vi "Next Column (name).vi"(8 "error in (no error)":errorcluster, 10 "parameter name":string, 11 "SQL Statement in":refnum<class "SQL Statement.lvclass">) -> (0 "error out":errorcluster, 3 "SQL Statement out":refnum<class "SQL Statement.lvclass">)   [LabVIEW 2023]
doc: "Sets the next parameter to be bound to, by its name. Name formats are ?NNN, :VVV, @VVV or $VVV where NNN are numeric digits and VVV are alphanumeric characters. Names are specified in the SQL statement."
uses:
  SQL Statement.lvclass
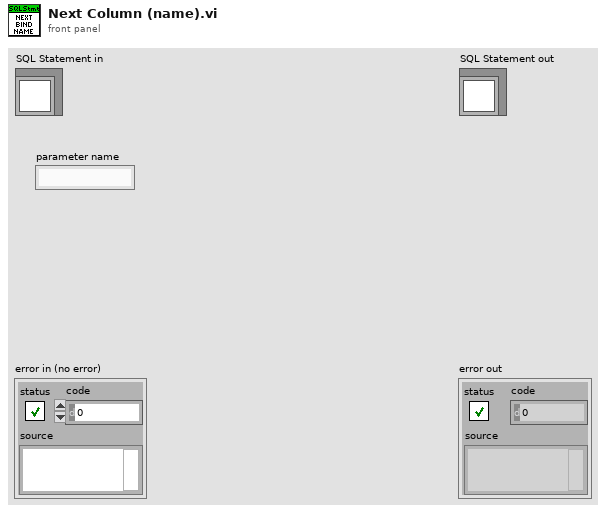
[diagram p1: front panel]
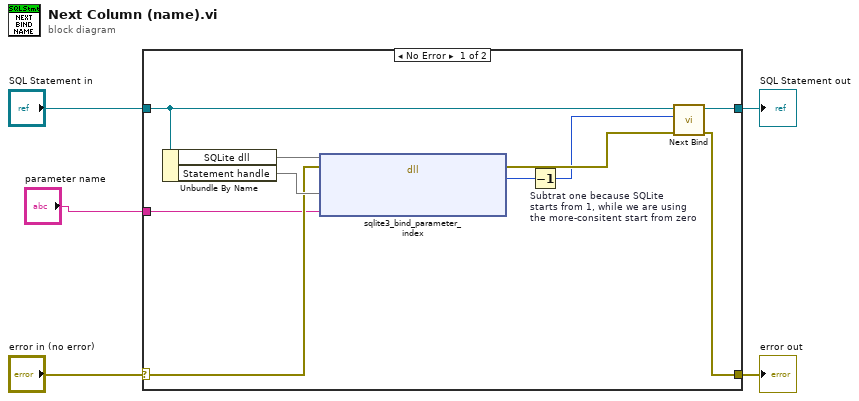
[diagram p0: block diagram]
diagram:
  n1 = case shown="No Error" "error in (no error)" {
    selector: "error in (no error)" -> [w13 w17]
    tunnel: [w7 w17] -> w4
    tunnel: [w10 w16] -> w2
    tunnel: "SQL Statement in" -> [w11 w16]
    tunnel: "parameter name" -> [w12 _]
    frame No Error {
      n2 = Unbundle By Name(w11) -> ("SQLite dll"=w15, "Statement handle"=w14)
      n3 = dll-call lib="C:/LabVIEW_JDP/Support/SQLite/sqlite3.dll" fn="sqlite3_bind_parameter_index"(path in=w15, error in=w13, "Statement"=w14, "name"=w12) -> (error out=w8:errorcluster, "Paramter index"=w9:i32)  [unwired: 3 in, 1 out]
      n4 = Decrement "Subtrat one because SQLite\nstarts from 1, while we are using\nthe more-consitent start from zero"(x=w9) -> (x-1=w6:i32)
      n5 = call "Next Bind.vi"("error in (no error)"=w8, "Next Bind"=w6, "SQL Statement in"=w11) -> ("error out"=w7:errorcluster, "SQL Statement out"=w10:refnum<class "SQL Statement.lvclass">)  [unwired: 7 in]
    }
    frame Error {
    }
  }
  "error out" <- w4
  "SQL Statement out" <- w2
